vi "mouseTest.vi"() -> ()   [LabVIEW 2010]
panel:
  out "Waveform Graph":dynamicdata(graph)
  out "HR 2":dbl
  in  "stop":bool
  in  "VISA Resource Name":refnum<visa-resource-name>
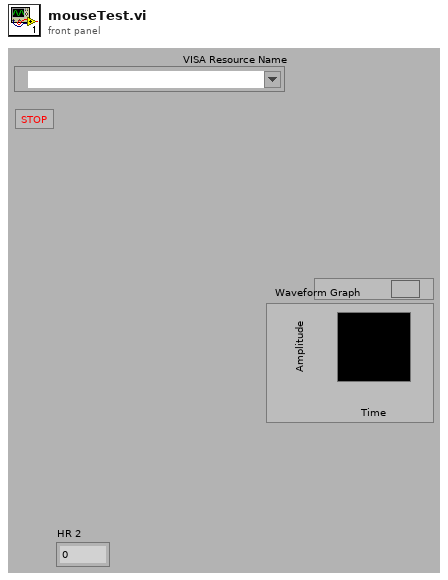
[diagram p1: front panel]
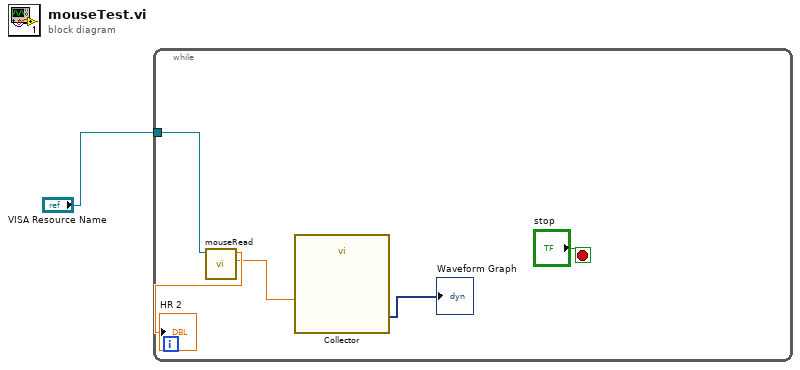
[diagram p0: block diagram]
diagram:
  n1 = while {
    tunnel: "VISA Resource Name" -> [w2]
    stop <- "stop" stop-if-true
    n2 = call "mouseRead.vi"("VISA Resource Name"=w2) -> ("Signal"=w4:dbl, "Times"=→"HR 2":dbl)  [unwired: 9 in]
    n3 = call "Collector"("Signals"=w4) -> ("Collected Signals"=→"Waveform Graph":dynamicdata)  [unwired: 9 in, 1 out]
  }
